vi "mainPanel.vi"() -> ()   [LabVIEW 2024]
uses:
  <vilib>/Math Plots/3D Math Plots/3D Pie/3D Pie XCtrl/3D Pie.xctl
  <vilib>/Math Plots/3D Math Plots/3D Pie/3D Pie Datatype/Public/Plot Helper (Vector).vi
  <vilib>/Math Plots/3D Math Plots/3D Pie/3D Pie Datatype/3D Pie Datatype.lvclass
panel:
  in  "Tab D":bool
  in  "Tab C":bool
  in  "Tab B":bool
  in  "Tab A":bool
  out "Abort":bool
  in  "Tab Control":enum32{"A", "B", "B 2", "B 3"}(tab)
  out "Image":T1(plugin-control)
  out "Nombre de véhicules:":dbl
  out "Nombre de \nvéhicules suspects:":dbl
  out "Localisation":string
  out "Date":string
  out "Nombre de véhicules Total":string
  out "Nombre véhicules Suspects":string
  out "Taux d'embouteillage":dbl(knob) scale=0.0..100.0
  out "Horaire":string[](array[string])
  out "Immatricule":string[](array[string])
  out "Dernière Alerte de suspection":string
  out "new picture 2":picture
  out "Nombre de véhicules Total":refnum<class "3D Plot Datatype.lvclass">[](xcontrol)
  out "String":string
  out "String 2":string
  in  "Quit":bool
  # "DIRECT"
  # "BILAN"
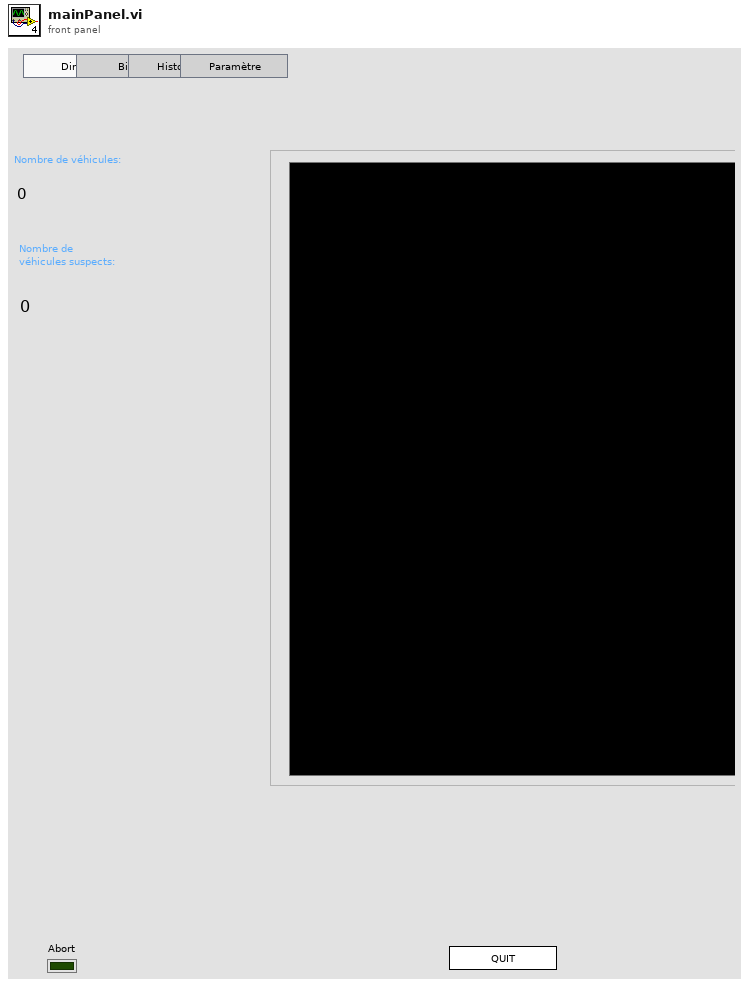
[diagram p1: front panel]
types:
  T1 = typedef "IMAQ Image.ctl" = refnum<image>
  T2 = cluster{"Foreground Color":u32, "Background Color":u32}
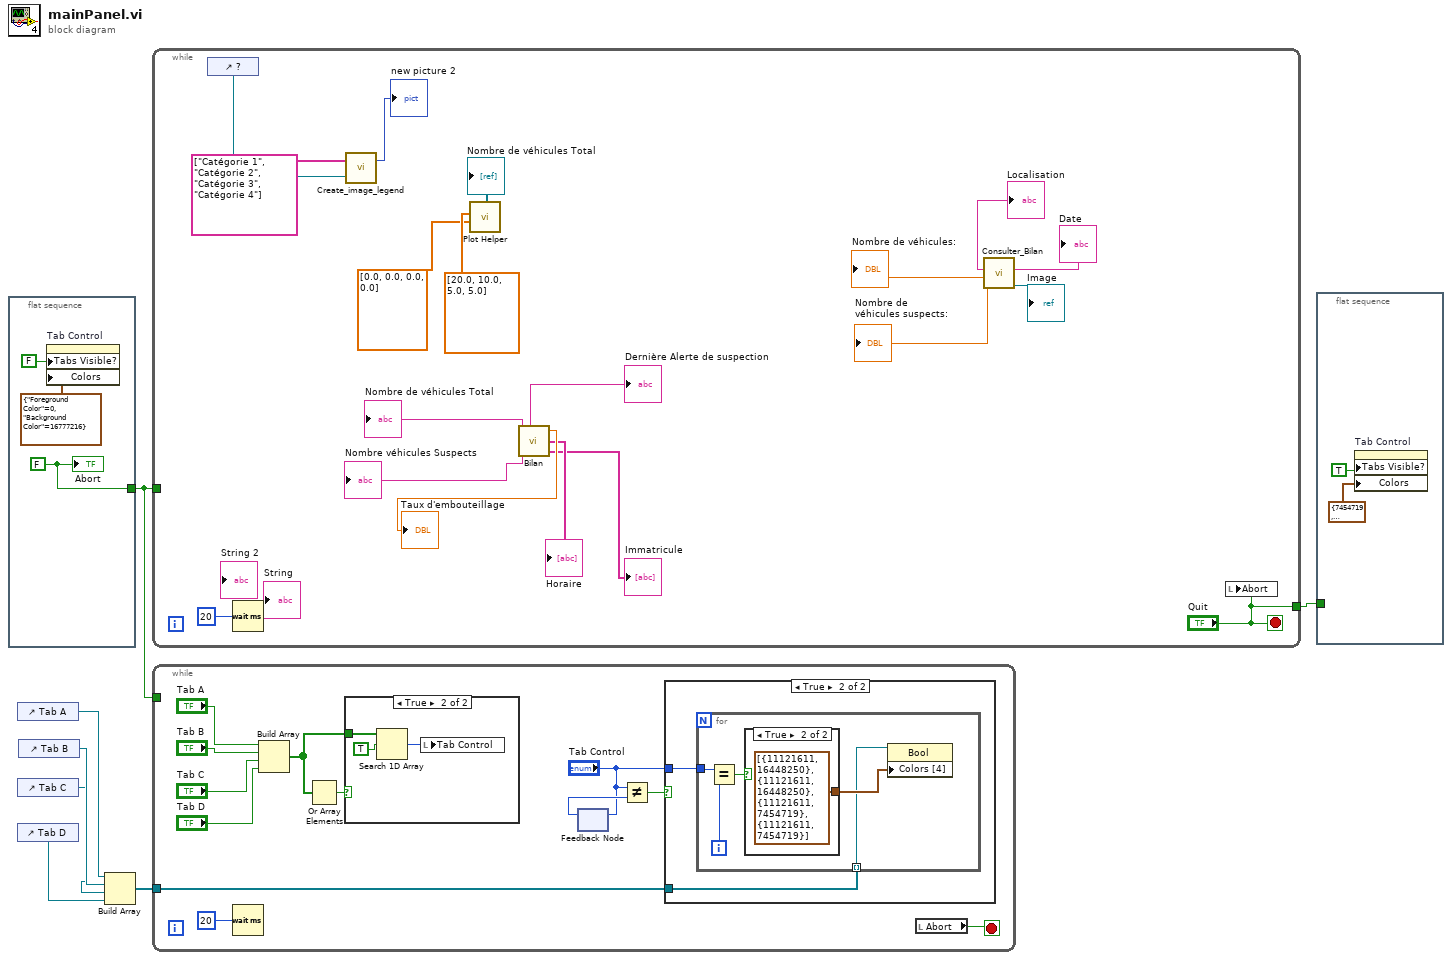
[diagram p0: block diagram]
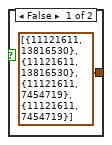
[diagram p3: hidden frame]
diagram:
  n1 = flat-sequence {
    tunnel: [w10] -> w7
    frame #0 {
      w10 = FALSE ("Abort")
      n2 = property on="Tab Control" class="TabCtl (strict)"("Tabs Visible?"=FALSE ("Visible"), "Colors"=T2 {"Foreground Color"=0, "Background Color"=16777216}) -> ()  [unwired: 2 in, 2 out]
      "Abort" <- w10
    }
  }
  n3 = control-ref of="Tab A"() -> (w4:refnum<vi>)
  n4 = control-ref of="Tab C"() -> (w2:refnum<vi>)
  n5 = control-ref of="Tab D"() -> (w1:refnum<vi>)
  n6 = control-ref of="Tab B"() -> (w3:refnum<vi>)
  n7 = Build Array(w4, w3, w2, w1) -> (w6:refnum<vi>[])
  n8 = while {
    tunnel: w7 -> [_]
    tunnel: ["Quit"] -> w5
    stop <- "Quit" stop-if-true
    n9 = control-ref of="?"() -> (w17:refnum<vi>)
    n10 = Wait (ms)(milliseconds to wait=u32 20) -> ()  [unwired: 1 out]
    n11 = call "Create_image_legend.vi"("Nombre de véhicules Total 2"=w17, "Immatricule"=string[] ["Catégorie 1", "Catégorie 2", "Catégorie 3", "Catégorie 4"]) -> ("new picture"=→"new picture 2":picture)  [unwired: 1 in]
    n12 = call-poly <vilib>:"Plot Helper.vi"("offset vector"=dbl[] [0.0, 0.0, 0.0, 0.0], "x vector"=dbl[] [20.0, 10.0, 5.0, 5.0]) -> ("3D Plot lvclass Array out"=→"Nombre de véhicules Total":refnum<class "3D Plot Datatype.lvclass">[])  [unwired: 1 in, 8 out]
    n13 = call "Bilan.vi"() -> ("Nombre de véhicules Total"=→"Nombre de véhicules Total":string, "Nombre véhicules Suspects"=→"Nombre véhicules Suspects":string, "Dernière Alerte de suspection"=→"Dernière Alerte de suspection":string, "Taux d'embouteillage"=→"Taux d'embouteillage":dbl, "Horaire"=→"Horaire":string[], "Immatricule"=→"Immatricule":string[])  [unwired: 2 in]
    n14 = call "Consulter_Bilan.vi"() -> ("Date"=→"Localisation":string, "Nombre de véhicules:"=→"Nombre de véhicules:":dbl, "Nombre de \nvéhicules suspects:"=→"Nombre de \nvéhicules suspects:":dbl, "Localisation"=→"Date":string, "Image"=→"Image":T1)  [unwired: 6 in]
    n15 = local write "Abort"("Quit") -> ()
  }
  n16 = while {
    tunnel: w7 -> [_]
    tunnel: w6 -> [w36]
    stop <- w41 stop-if-true
    n17 = Wait (ms)(milliseconds to wait=u32 20) -> ()  [unwired: 1 out]
    n18 = Build Array("Tab A", "Tab B", "Tab C", "Tab D") -> (w34:bool[])
    n19 = Or Array Elements(Boolean array=w34) -> (logical OR=w35:bool)
    n20 = case shown="True" w35 {
      tunnel: w34 -> [_ w51]
      frame False {
      }
      frame True {
        n21 = Search 1D Array(1D array=w51, element=TRUE) -> (index of element=w52:i32)  [unwired: 1 in]
        n22 = local write "Tab Control"(w52) -> ()
      }
    }
    n23 = feedback-in #1("Tab Control") -> ()
    n24 = feedback #1() -> (w38:enum32{"A", "B", "B 2", "B 3"})  [unwired: 1 in]
    n25 = Not Equal?(x="Tab Control", y=w38) -> (x != y?=w39:bool)
    n26 = case shown="True" w39 {
      tunnel: "Tab Control" -> [_ w43]
      tunnel: w36 -> [_ w42]
      frame False {
      }
      frame True {
        n27 = for {
          tunnel: w43 -> [w46]
          tunnel: w42 -> [w44] mode=indexing
          i -> [w47]
          n28 = Equal?(x=w46, y=w47) -> (x = y?=w48:bool)
          n29 = case shown="True" w48 {
            tunnel: [cluster{u32, u32}[] [{11121611, 13816530}, {11121611, 13816530}, {11121611, 7454719}, {11121611, 7454719}] ("Colors [4]") cluster{u32, u32}[] [{11121611, 16448250}, {11121611, 16448250}, {11121611, 7454719}, {11121611, 7454719}] ("Colors [4]")] -> w45
            frame False {
            }
            frame True {
            }
          }
          n30 = property class="Bool"(reference=w44, "Colors [4]"=w45) -> ()  [unwired: 1 in, 2 out]
        }
      }
    }
    n31 = local read "Abort"() -> (w41:bool)
  }
  n32 = flat-sequence {
    tunnel: w5 -> [_]
    frame #0 {
      n33 = property on="Tab Control" class="TabCtl (strict)"("Tabs Visible?"=TRUE ("Visible"), "Colors"=T2 {"Foreground Color"=7454719, "Background Color"=7454719}) -> ()  [unwired: 2 in, 2 out]
    }
  }
